vi "Cleanup.vi"(8 "error in (no error)":errorcluster, 11 "GCentral API in":refnum<class "GCentral API.lvclass">) -> (0 "error out":errorcluster)   [LabVIEW 2020, in "GCentral-API.lvlib" / "GCentral API.lvclass"]
uses:
  GCentral API.lvclass
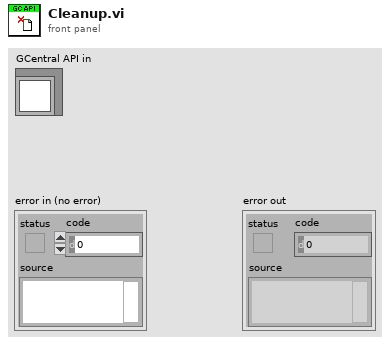
[diagram p1: front panel]
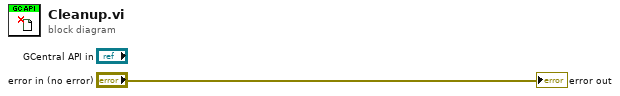
[diagram p0: block diagram]
diagram:
  "error out" <- "error in (no error)"
